vi "Pressure Scan Compute.vi"(8 "error in":errorcluster, 10 "Pressure U":waveform(dbl)[](array[waveform]), 11 "Water Tunnel Results in":refnum<class "Water Tunnel Results.lvclass">) -> (0 "error out":errorcluster, 2 "Pressure":waveform(dbl)[](array[waveform]), 3 "Water Tunnel Results out":refnum<class "Water Tunnel Results.lvclass">)   [LabVIEW 2019, in "Results.lvlib" / "Water Tunnel Results.lvclass"]
uses:
  Water Tunnel Results.lvclass
  Water Tunnel Results.lvclass/Water Tunnel Results.ctl
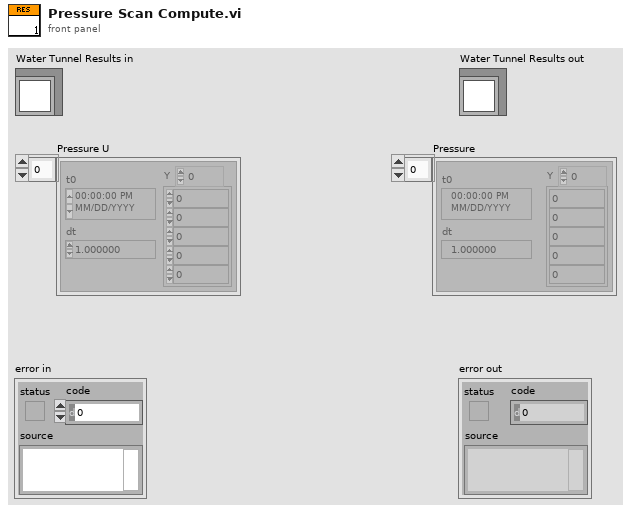
[diagram p1: front panel]
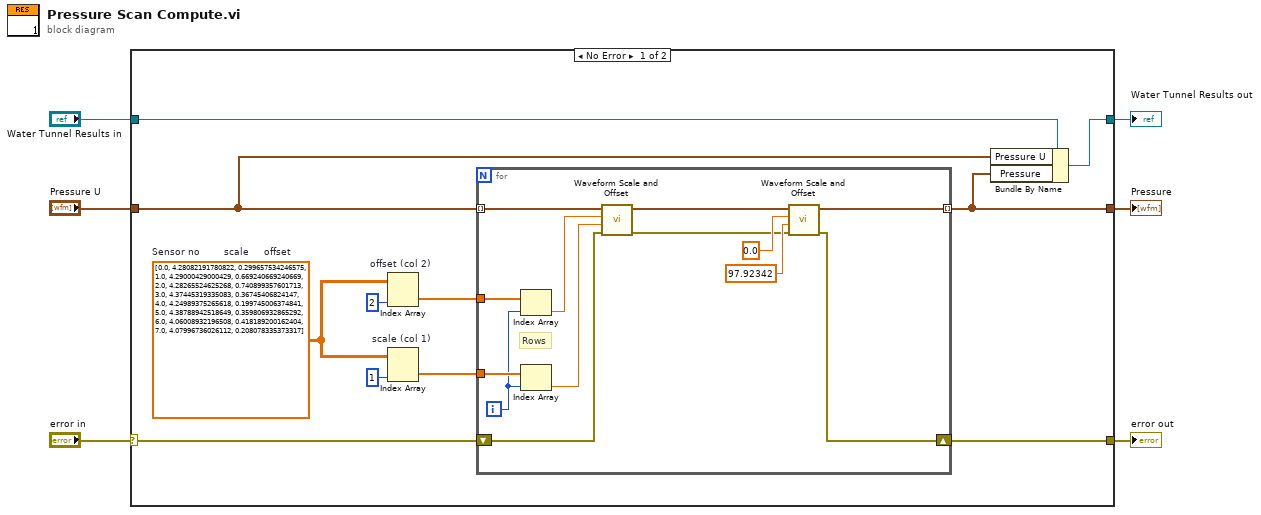
[diagram p0: block diagram]
diagram:
  n1 = case shown="No Error" "error in" {
    selector: "error in" -> [w8 w32]
    tunnel: [w7 w32] -> w5
    tunnel: [w16 w31] -> w3
    tunnel: "Water Tunnel Results in" -> [w17 w31]
    tunnel: "Pressure U" -> [w15 _]
    tunnel: [w14 _] -> w1
    frame No Error {
      w11 = dbl[][] [[0.0, 4.28082191780822, 0.299657534246575], [1.0, 4.29000429000429, 0.669240669240669], [2.0, 4.28265524625268, 0.740899357601713], [3.0, 4.37445319335083, 0.36745406824147], [4.0, 4.24989375265618, 0.199745006374841], [5.0, 4.38788942518649, 0.359806932865292], [6.0, 4.06008932196508, 0.418189200162404], [7.0, 4.07996736026112, 0.208078335373317]]  # Sensor no        scale     offset
      n2 = Index Array "offset (col 2)"(array=w11, index (col)=2 ("disabled index (col)")) -> (element=w10:dbl[])  [unwired: 1 in]
      n3 = Index Array "scale (col 1)"(array=w11, index (col)=1 ("disabled index (col)")) -> (element=w9:dbl[])  [unwired: 1 in]
      n4 = for {
        tunnel: w15 -> [w30] mode=indexing
        tunnel: [w23] -> w14 mode=indexing
        tunnel: w10 -> [w29]
        tunnel: w9 -> [w28]
        shift-right: [w18] -> w7
        shift-left: w8 -> [w20]
        i -> [w27]
        # "Rows"
        n5 = Index Array(array=w29, index=w27) -> (element=w25:dbl)
        n6 = Index Array(array=w28, index=w27) -> (element=w26:dbl)
        n7 = call <vilib>:"Waveform Scale and Offset.vi"("error in (no error)"=w20, "scale"=w26, "offset"=w25, "waveform in"=w30) -> ("error out"=w19:errorcluster, "waveform out"=w24:waveform(dbl))  [unwired: 6 in]
        n8 = call <vilib>:"Waveform Scale and Offset.vi"("error in (no error)"=w19, "scale"=97.92342, "offset"=0.0, "waveform in"=w24) -> ("error out"=w18:errorcluster, "waveform out"=w23:waveform(dbl))  [unwired: 6 in]
      }
      n9 = Bundle By Name(cluster=w17, "Pressure U"=w15, "Pressure"=w14) -> (w16:refnum<class "Water Tunnel Results.lvclass">)
    }
    frame Error {
    }
  }
  "error out" <- w5
  "Water Tunnel Results out" <- w3
  "Pressure" <- w1
